vi "ConvertDcafStepStatus.vi"(11 "DCAF Step State":T2) -> (3 "Systemlink Status":T1=enum."None")   [LabVIEW 2018, in "TestMonitor.lvclass"]
doc: "This VI converts the DCAF Step State into the Systemlink Step Status"
uses:
  TestMonitor.lvclass
  Step/Execution/Step Status.ctl
  <vilib>/Skyline/TestMonitor/Shared/typedefs/Status Type.ctl
  <vilib>/Skyline/TestMonitor/Shared/NI SystemLink Test Monitor.lvlib
  Step/Execution/Step.lvclass
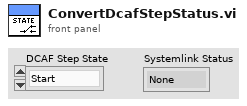
[diagram p1: front panel]
types:
  T1 = typedef "NI SystemLink Test Monitor.lvlib/Status Type.ctl" = enum16{"Failed", "Passed", "Looping", "Skipped", "Custom", "Done", "Running", "Waiting", "Terminated", "Errored", "Timed Out", "None"}
  T2 = typedef "Step.lvclass/Step Status.ctl" = enum16{"Start", "Passed", "Failed", "Error", "Done", "Terminated", "Skipped", "Running"}
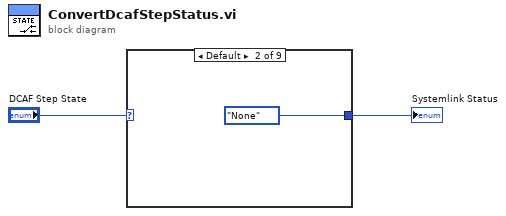
[diagram p0: block diagram]
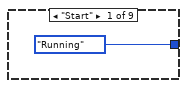
[diagram p2: hidden frame]
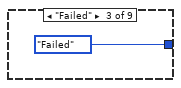
[diagram p3: hidden frame]
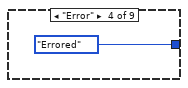
[diagram p4: hidden frame]
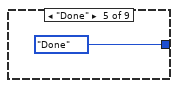
[diagram p5: hidden frame]
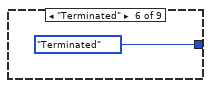
[diagram p6: hidden frame]
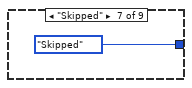
[diagram p7: hidden frame]
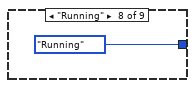
[diagram p8: hidden frame]
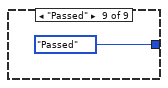
[diagram p9: hidden frame]
diagram:
  n1 = case shown="Default" "DCAF Step State" {
    tunnel: [Status_Type."Running" ("Systemlink Status") Status_Type."None" ("Systemlink Status") Status_Type."Failed" ("Systemlink Status") Status_Type."Errored" ("Systemlink Status") Status_Type."Done" ("Systemlink Status") Status_Type."Terminated" ("Systemlink Status") Status_Type."Skipped" ("Systemlink Status") Status_Type."Running" ("Systemlink Status") Status_Type."Passed" ("Systemlink Status")] -> w1
    frame "Start" {
    }
    frame Default {
    }
    frame "Failed" {
    }
    frame "Error" {
    }
    frame "Done" {
    }
    frame "Terminated" {
    }
    frame "Skipped" {
    }
    frame "Running" {
    }
    frame "Passed" {
    }
  }
  "Systemlink Status" <- w1
